vi "Test.vi"   [LabVIEW 2013]
doc: "This VI is called when test mode begins, and will automatically be terminated when it ends. You can add manual or automatic tests and invoke them from the dashboard."
uses:
  Robot Global Data.vi
  <vilib>/Rock Robotics/WPI/MotorControl/WPI_MotorControlOpenCANJaguar.vi
types:
  T1 = typedef "WPI_MotorControlDeviceRef.ctl" = cluster{"DeviceStatus":errorcluster, "Type":enum16{"PWM", "CAN"}, "PWM":cluster{"Digital Module":T2, "PWM Channel":T3, "DeadBand":T4}, "CAN":cluster{"Device Number":u8, "Control Mode":T5, "Semaphore":T6, "Max Vout":dbl}, "Invert":bool, "TransformRef":T7, "InvTransformRef":T7}
  T2 = typedef "FPGA_TypedefDigitalModule.ctl" = enum16{"Digital Module 1", "Digital Module 2"}
  T3 = typedef "FPGA_DIOPWMChannel.ctl" = enum8{"PWM 1", "PWM 2", "PWM 3", "PWM 4", "PWM 5", "PWM 6", "PWM 7", "PWM 8", "PWM 9", "PWM 10", "Invalid"}
  T4 = typedef "WPI_PWMDeadband.ctl" = cluster{"Name":string, "maxPositivePwm":i32, "minPositivePwm":i32, "centerPwm":i32, "maxNegativePwm":i32, "minNegativePwm":i32, "angularRange":u16}
  T5 = typedef "WPI_CANJaguar_ControlMode.ctl" = enum8{"Percent VBus", "Current", "Speed", "Position", "Voltage"}
  T6 = typedef "Semaphore RefNum" = refnum<k1>
  T7 = typedef "WPI_PWMTransform_ConPane.ctl" = refnum<vi>
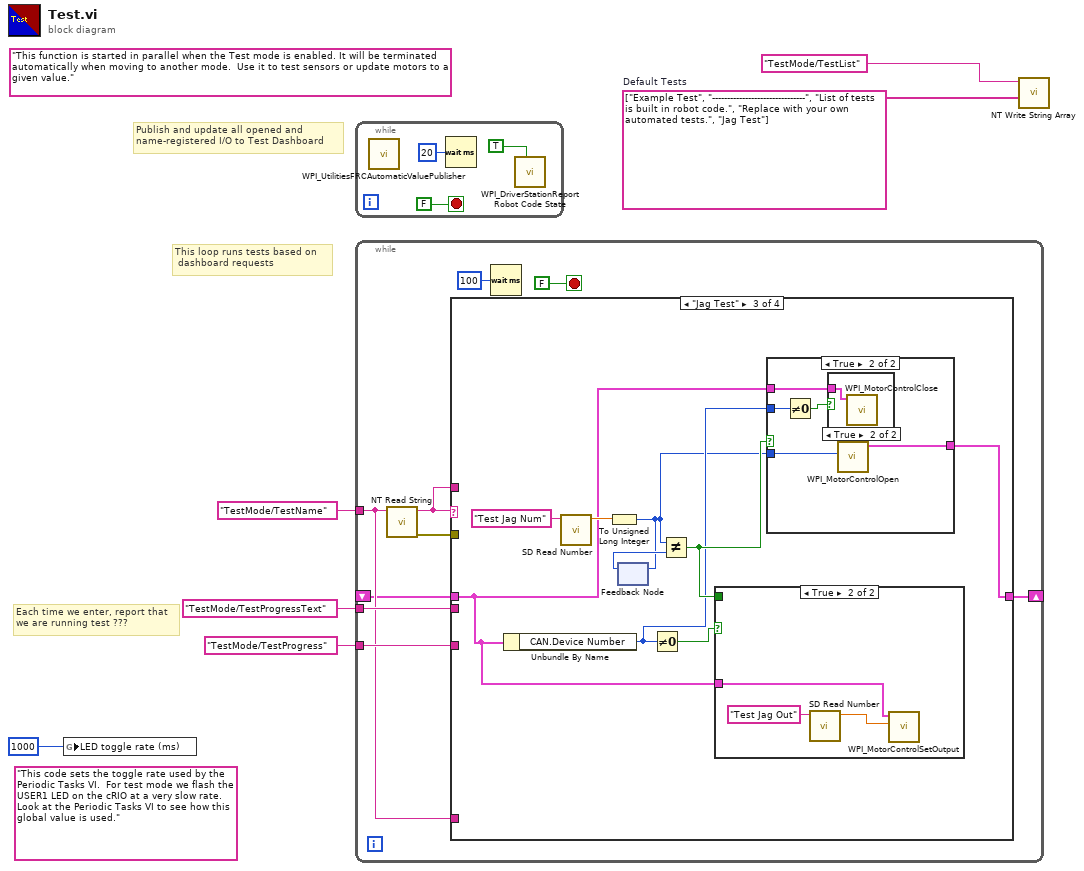
[diagram p0: block diagram]
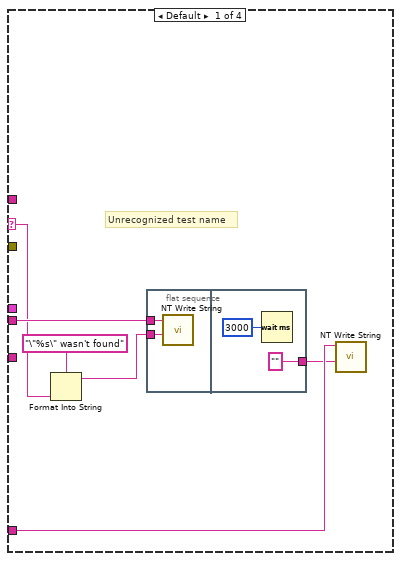
[diagram p2: hidden frame]
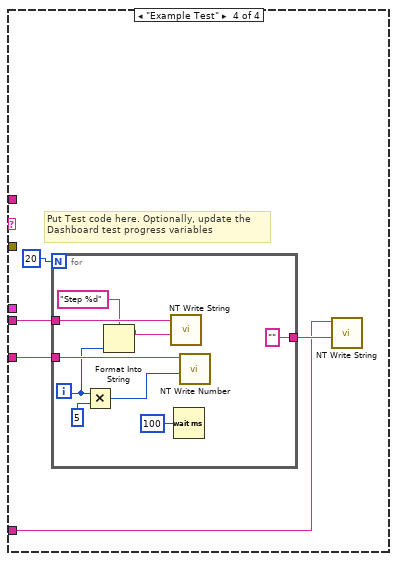
[diagram p7: hidden frame]
diagram:
  w2 = string[] ["Example Test", "-------------------------------", "List of tests is built in robot code.", "Replace with your own automated tests.", "Jag Test"]  # Default Tests
  (unwired) "This code sets the toggle rate used by the Periodic Tasks VI.  For test mode we flash the USER1 LED on the cRIO at a very slow rate.  Look at the Periodic Tasks VI to see how this global value is used."
  (unwired) "This function is started in parallel when the Test mode is enabled. It will be terminated automatically when moving to another mode.  Use it to test sensors or update motors to a given value."
  # "This loop runs tests based on \n dashboard requests"
  # "Publish and update all opened and\nname-registered I/O to Test Dashboard"
  # "Each time we enter, report that\nwe are running test ???"
  n1 = global write "Robot Global Data.vi" "LED toggle rate (ms)"(u32 1000 ("LED ms toggle rate")) -> ()
  n2 = while {
    stop <- FALSE stop-if-true
    n3 = call <vilib>:"WPI_UtilitiesFRCAutomaticValuePublisher.vi"() -> ()  [unwired: 12 in]
    n4 = Wait (ms)(milliseconds to wait=u32 20) -> ()  [unwired: 1 out]
    n5 = call <vilib>:"WPI_DriverStationReport Robot Code State.vi"("Test"=TRUE ("Autonomous")) -> ()  [unwired: 10 in, 1 out]
  }
  n6 = while {
    tunnel: "TestMode/TestName" ("Name") -> [w13]
    tunnel: "TestMode/TestProgressText" ("Name") -> [w16]
    tunnel: "TestMode/TestProgress" ("Name") -> [w15]
    shift-right: [w10] -> _
    shift-left: _ -> [w11]
    stop <- FALSE stop-if-true
    n7 = call <vilib>:"NT Read String.vi"("Name"=w13) -> ("error out"=w12:errorcluster, "String"=w14:string)  [unwired: 9 in]
    n8 = case shown="\"Jag Test\"" w14 {
      selector: w14 -> [w23 _ _ _]
      tunnel: w13 -> [w20 _ _ w48]
      tunnel: w16 -> [w24 _ _ w51]
      tunnel: w15 -> [_ _ _ w52]
      tunnel: w14 -> [_ _ _ _]
      tunnel: w12 -> [_ _ _ _]
      tunnel: w11 -> [_ _ w30 _]
      tunnel: [_ _ w31 _] -> w10
      frame Default {
        # "Unrecognized test name"
        n9 = Format Into String(format string="\"%s\" wasn't found" ("Name"), w23) -> (resulting string=w22:string)  [unwired: 2 in, 1 out]
        n10 = flat-sequence {
          tunnel: w24 -> [w25]
          tunnel: w22 -> [w26]
          tunnel: ["" ("Name")] -> w19
          frame #0 {
            n11 = call <vilib>:"NT Write String.vi"("String"=w26, "Name"=w25) -> ()  [unwired: 9 in, 1 out]
          }
          frame #1 {
            n12 = Wait (ms)(milliseconds to wait=u32 3000) -> ()  [unwired: 1 out]
          }
        }
        n13 = call <vilib>:"NT Write String.vi"("String"=w19, "Name"=w20) -> ()  [unwired: 9 in, 1 out]
      }
      frame "" {
        # "No test to run"
      }
      frame "Jag Test" {
        n14 = Unbundle By Name(w30) -> ("CAN.Device Number"=w32:u8)
        n15 = call <vilib>:"SD Read Number.vi"("Name"="Test Jag Num") -> ("Numeric"=w37:dbl)  [unwired: 8 in, 2 out]
        n16 = To Unsigned Long Integer(number=w37) -> (unsigned 32bit integer=w29:u32)
        n17 = feedback-in #1(w29) -> ()
        n18 = feedback #1() -> (w35:u32)  [unwired: 1 in]
        n19 = Not Equal To 0?(x=w32) -> (x != 0?=w34:bool)
        n20 = Not Equal?(x=w29, y=w35) -> (x != y?=w33:bool)
        n21 = case shown="True" w34 {
          tunnel: w33 -> [_ _]
          tunnel: w30 -> [_ w45]
          frame False {
          }
          frame True {
            n22 = call <vilib>:"SD Read Number.vi"("Name"="Test Jag Out") -> ("Numeric"=w46:dbl)  [unwired: 8 in, 2 out]
            n23 = call <vilib>:"WPI_MotorControlSetOutput.vi"("Output"=w46, "MotorControlDevRef"=w45) -> ()  [unwired: 7 in, 3 out]
          }
        }
        n24 = case shown="True" w33 {
          tunnel: [w38 w43] -> w31
          tunnel: w32 -> [_ w40]
          tunnel: w30 -> [w38 w41]
          tunnel: w29 -> [_ w39]
          frame False {
          }
          frame True {
            n25 = Not Equal To 0?(x=w40) -> (x != 0?=w42:bool)
            n26 = case shown="True" w42 {
              tunnel: w41 -> [_ w44]
              frame False {
              }
              frame True {
                n27 = call <vilib>:"WPI_MotorControlClose.vi"("MotorControlDevRef"=w44) -> ()  [unwired: 10 in, 1 out]
              }
            }
            n28 = call-poly <vilib>:"WPI_MotorControlOpen.vi"("Device Number"=w39) -> ("MotorControlDeviceRef"=w43:T1)  [unwired: 9 in, 1 out]
          }
        }
      }
      frame "Example Test" {
        # "Put Test code here. Optionally, update the\nDashboard test progress variables"
        n29 = for {
          N: 20 -> [_]
          tunnel: w52 -> [w61]
          tunnel: w51 -> [w59]
          tunnel: ["" ("String")] -> w49
          i -> [w56]
          n30 = Multiply(x=w56, y=u32 5 ("milliseconds to wait")) -> (x*y=w57:u32)
          n31 = Format Into String(format string="Step %d", w56) -> (resulting string=w54:string)  [unwired: 2 in, 1 out]
          n32 = call <vilib>:"NT Write String.vi"("String"=w54, "Name"=w59) -> ()  [unwired: 9 in, 1 out]
          n33 = Wait (ms)(milliseconds to wait=u32 100) -> ()  [unwired: 1 out]
          n34 = call <vilib>:"NT Write Number.vi"("Numeric"=w57, "Name"=w61) -> ()  [unwired: 9 in, 1 out]
        }
        n35 = call <vilib>:"NT Write String.vi"("String"=w49, "Name"=w48) -> ()  [unwired: 9 in, 1 out]
      }
    }
    n36 = Wait (ms)(milliseconds to wait=u32 100) -> ()  [unwired: 1 out]
  }
  n37 = call <vilib>:"NT Write String Array.vi"("String Array"=w2, "Name"="TestMode/TestList") -> ()  [unwired: 9 in, 1 out]
